vi "CRYSingleSineStep.vi"(0 "Fs":dbl=44100.0 format="%.2f", 1 "Freq":dbl=1000.0 format="%.2f", 2 "Cycles per freq":dbl=13.0 format="%.2f", 3 "Cycles discarded":dbl=1.0 format="%.2f", 4 "StartPhase":dbl format="%.2p") -> (5 "RelFreq":dbl=0.022675736961451247 format="%.2p", 6 "StopPhase":dbl format="%.2f", 7 "TotalSamples":i32=573, 8 "DiscardSamples":i32=44, 9 "ExtractSamples":i32=529, 10 "TimeCorrection":dbl=-0.0008163265306122299 format="%.5p")   [LabVIEW 2013]
panel:
  out "ActDiscCycles":dbl=1.0 format="%.2f"
  out "ActTotCycles":dbl=13.0 format="%.2f"
  out "DeltaPhase":dbl=8.16326530612245 format="%.2p"
  out "PhaseCorrection":dbl=-0.8163265306122298 format="%.2p"
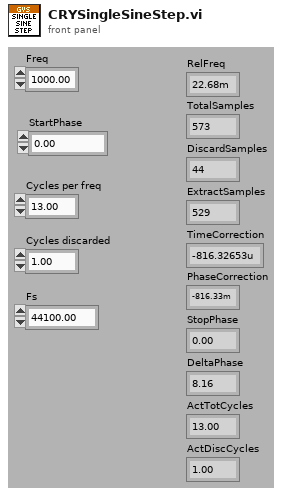
[diagram p1: front panel]
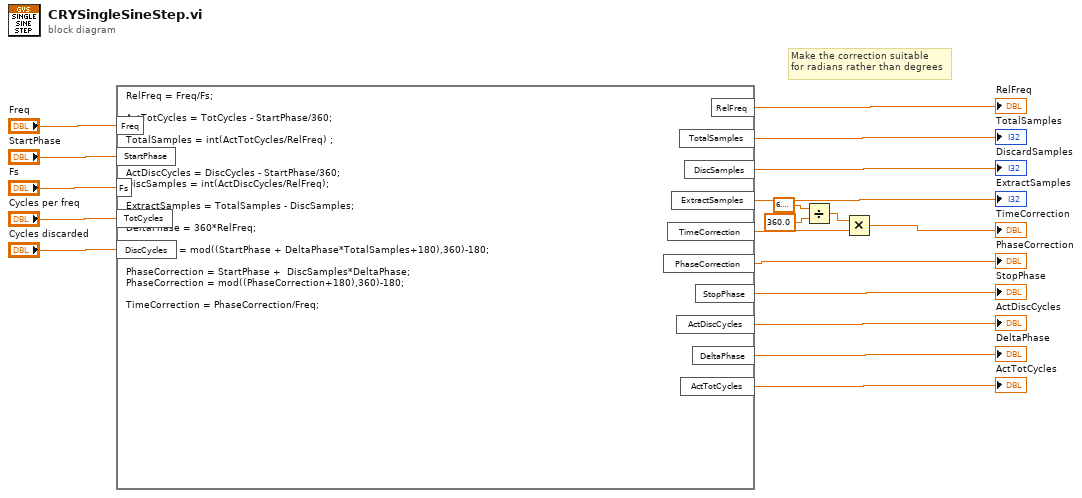
[diagram p0: block diagram]
diagram:
  # "Make the correction suitable \nfor radians rather than degrees"
  n1 = formula code="RelFreq = Freq/Fs;\n\nActTotCycles = TotCycles - StartPhase/360;\n\nTotalSamples = int(ActTotCycles/RelFreq) ;\n\n\nActDiscCycles = DiscCycles - StartPhase/360;\nDiscSamples = int(ActDiscCycles/RelFreq);\n\nExtractSamples = TotalSamples - DiscSamples;\n\nDeltaPhase = 360*RelFreq;\n\nStopPhase = mod((StartPhase + DeltaPhase*TotalSamples+180),360)-180;\n\nPhaseCorrection = StartPhase +  DiscSamples*DeltaPhase;\nPhaseCorrection = mod((PhaseCorrection+180),360)-180;\n\nTimeCorrection = PhaseCorrection/Freq;"("Freq"="Freq", "StartPhase"="StartPhase", "Fs"="Fs", "TotCycles"="Cycles per freq", "DiscCycles"="Cycles discarded") -> ("RelFreq"=→"RelFreq":dbl, "TotalSamples"=→"TotalSamples":dbl, "DiscSamples"=→"DiscardSamples":dbl, "ExtractSamples"=→"ExtractSamples":dbl, "TimeCorrection"=w2:dbl, "ActTotCycles"=→"ActTotCycles":dbl, "DeltaPhase"=→"DeltaPhase":dbl, "ActDiscCycles"=→"ActDiscCycles":dbl, "PhaseCorrection"=→"PhaseCorrection":dbl, "StopPhase"=→"StopPhase":dbl)
  n2 = Divide(x=6.283185307179586, y=360.0) -> (x/y=w1:dbl)
  n3 = Multiply(x=w1, y=w2) -> (x*y=→"TimeCorrection":dbl)
